vi "CalculateDelay2.vi"(8 "input valid":bool=TRUE, 9 "cos_fi":fxp<+/-,16,2>, 10 "sin fi":fxp<+/-,16,2>, 11 "Data in":fxp<+/-,16,14>[](array[numeric])=[0.0, 0.0, 0.0, 0.0]) -> (0 "output valid":bool, 3 "Data out":fxp<+/-,16,14>[](array[numeric]))   [LabVIEW 2013]
doc: "Calculates various combinations on I_in, Q_in and cos(fi) and sin(fi) to be used later to delay the output signal"
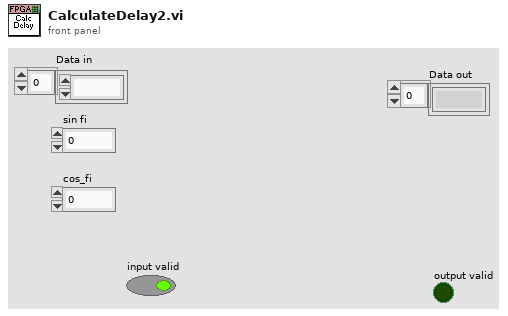
[diagram p1: front panel]
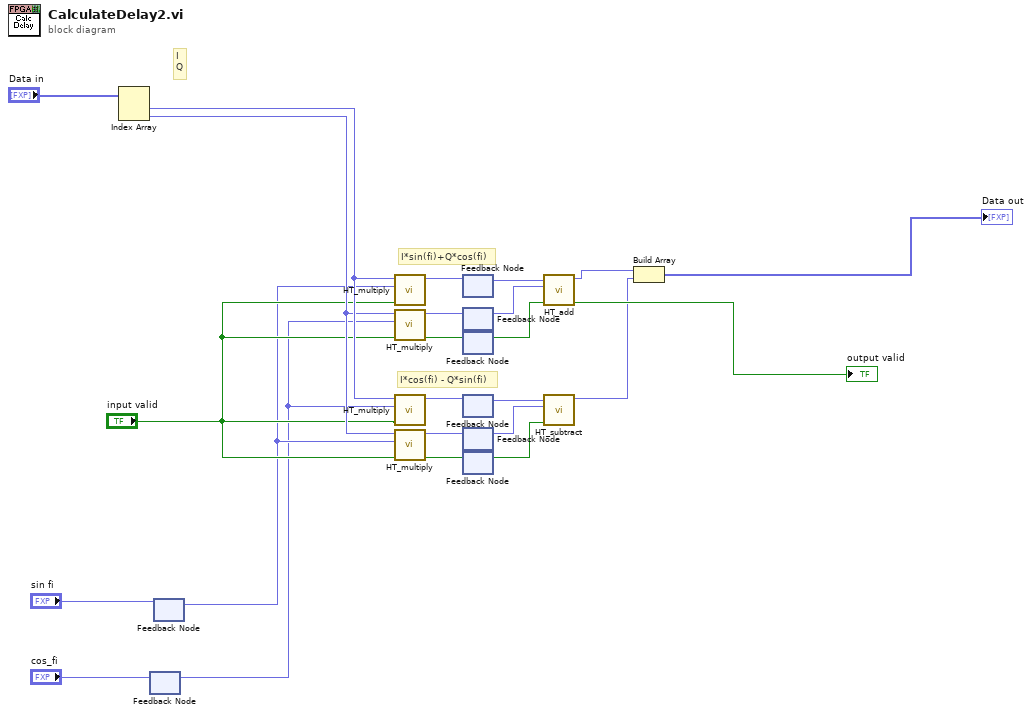
[diagram p0: block diagram]
diagram:
  # "I*cos(fi) - Q*sin(fi)"
  # "I\nQ"
  # "I*sin(fi)+Q*cos(fi)"
  n1 = Index Array(array="Data in") -> (element #1=w11:fxp<+/-,16,14>, element #2=w10:fxp<+/-,16,14>)  [unwired: 2 in]
  n2 = feedback #1() -> (w3:fxp<+/-,16,2>)  [unwired: 1 in]
  n3 = feedback-in #1("cos_fi") -> ()
  n4 = feedback #2() -> (w5:fxp<+/-,16,2>)  [unwired: 1 in]
  n5 = feedback-in #2("sin fi") -> ()
  n6 = call "HT_multiply.vi"("input valid"="input valid", "y"=w5, "x"=w11) -> ("x*y"=w23:fxp<+/-,16,14>)  [unwired: 7 in, 1 out]
  n7 = call "HT_multiply.vi"("input valid"="input valid", "y"=w3, "x"=w10) -> ("output valid"=w18:bool, "x*y"=w20:fxp<+/-,16,14>)  [unwired: 7 in]
  n8 = call "HT_multiply.vi"("input valid"="input valid", "y"=w3, "x"=w11) -> ("x*y"=w12:fxp<+/-,16,14>)  [unwired: 7 in, 1 out]
  n9 = call "HT_multiply.vi"("input valid"="input valid", "y"=w5, "x"=w10) -> ("output valid"=w17:bool, "x*y"=w15:fxp<+/-,16,14>)  [unwired: 7 in]
  n10 = feedback #3() -> (w22:fxp<+/-,16,14>)  [unwired: 1 in]
  n11 = feedback-in #3(w23) -> ()
  n12 = feedback #4() -> (w19:fxp<+/-,16,14>)  [unwired: 1 in]
  n13 = feedback-in #4(w20) -> ()
  n14 = feedback #5() -> (w21:bool)  [unwired: 1 in]
  n15 = feedback-in #5(w18) -> ()
  n16 = feedback #6() -> (w13:fxp<+/-,16,14>)  [unwired: 1 in]
  n17 = feedback-in #6(w12) -> ()
  n18 = feedback #7() -> (w16:fxp<+/-,16,14>)  [unwired: 1 in]
  n19 = feedback-in #7(w15) -> ()
  n20 = feedback #8() -> (w14:bool)  [unwired: 1 in]
  n21 = feedback-in #8(w17) -> ()
  n22 = call "HT_add.vi"("input valid"=w21, "y"=w19, "x"=w22) -> ("output valid"=→"output valid":bool, "x+y"=w2:fxp<+/-,16,14>)  [unwired: 7 in]
  n23 = call "HT_subtract.vi"("input valid"=w14, "y"=w16, "x"=w13) -> ("x+y"=w1:fxp<+/-,16,14>)  [unwired: 7 in, 1 out]
  n24 = Build Array(w2, w1) -> (→"Data out":fxp<+/-,16,14>[])
